vi "DataPropertyEnumToString.vi"(11 "property":T1) -> (3 "string":string)   [LabVIEW 2017, in "FileManager.lvlib"]
uses:
  <vilib>/addons/InsightCM/Devices/Shared/Common/FileManager/FileManager.lvlib
  <vilib>/addons/InsightCM/Devices/Shared/Common/FileManager/controls/DataPropertyNames.ctl
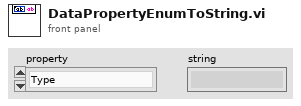
[diagram p1: front panel]
types:
  T1 = typedef "DataPropertyNames.ctl" = enum16{"Type", "EventRef", "FilePath", "DataGroup", "AcquisitionTimestamp", "StreamId", "StreamBlock", "TrendPointsOnly", "ExtraLargeFile"}
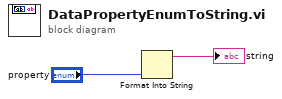
[diagram p0: block diagram]
diagram:
  n1 = Format Into String("property") -> (resulting string=→"string":string)  [unwired: 3 in, 1 out]
